vi "ProcCore.vi"(6 "SecondaryData Feed":refnum<queue>, 7 "ProcessParams":T1={"DisplayIncrement"=0, "DisplayIncrementRef"=refnum, "Rep .Rate (Hz)"=10.0, "Save"=FALSE, "SW_Average"=0, "Filter"=enum."None", "FilterParams"=variant, "DAQParams"={"TrigDelay"=0.0, "Offset"=0, "Resolution"=-32768, "Range (mV)"=0, "Sample Rate"=100000000.0, "Depth"=16384.0, "Segments"=1}, "Graph"=[], "CmdParams."=variant, "Average(SW)Ref"=refnum, "Calibr.Params"=refnum, "SignalSegmentRef"=refnum, "WriterQueue"=refnum, "SecData_Interpolation"=FALSE} {"DAQParams"."Segments" min=1 max=1024 step=1; "DAQParams"."Sample Rate" format="%.0p"}, 8 "error in":errorcluster, 9 "Signal buffer in":refnum<queue>, 10 "CtrlQueue in":refnum<queue>) -> (0 "error out":errorcluster)   [LabVIEW 2014]
uses:
  <instrlib>/GenericDAQ/VI/GenericDAQ_Signal.ctl
  ProcessParams.ctl
  ControlDef/ProcessingMode.ctl
  DAQParams.ctl
  DisplayGraph.ctl
  Binning/BinType.ctl
  ControlDef/Average#.ctl
  Files/Signal_Segment.ctl
  ControlDef/Signal.ctl
  ProcessStates.ctl
  <instrlib>/GenericMotionCore/Public/SecondaryDataFeed.ctl
  Binning/SpectrumBinning.vi
  MassResolutionCalc/FindMassResolution_Single.vi
  <instrlib>/GenericMotionCore/GenericMotionCore.lvlib
  <instrlib>/GenericDAQ/GenericDAQ.lvlib
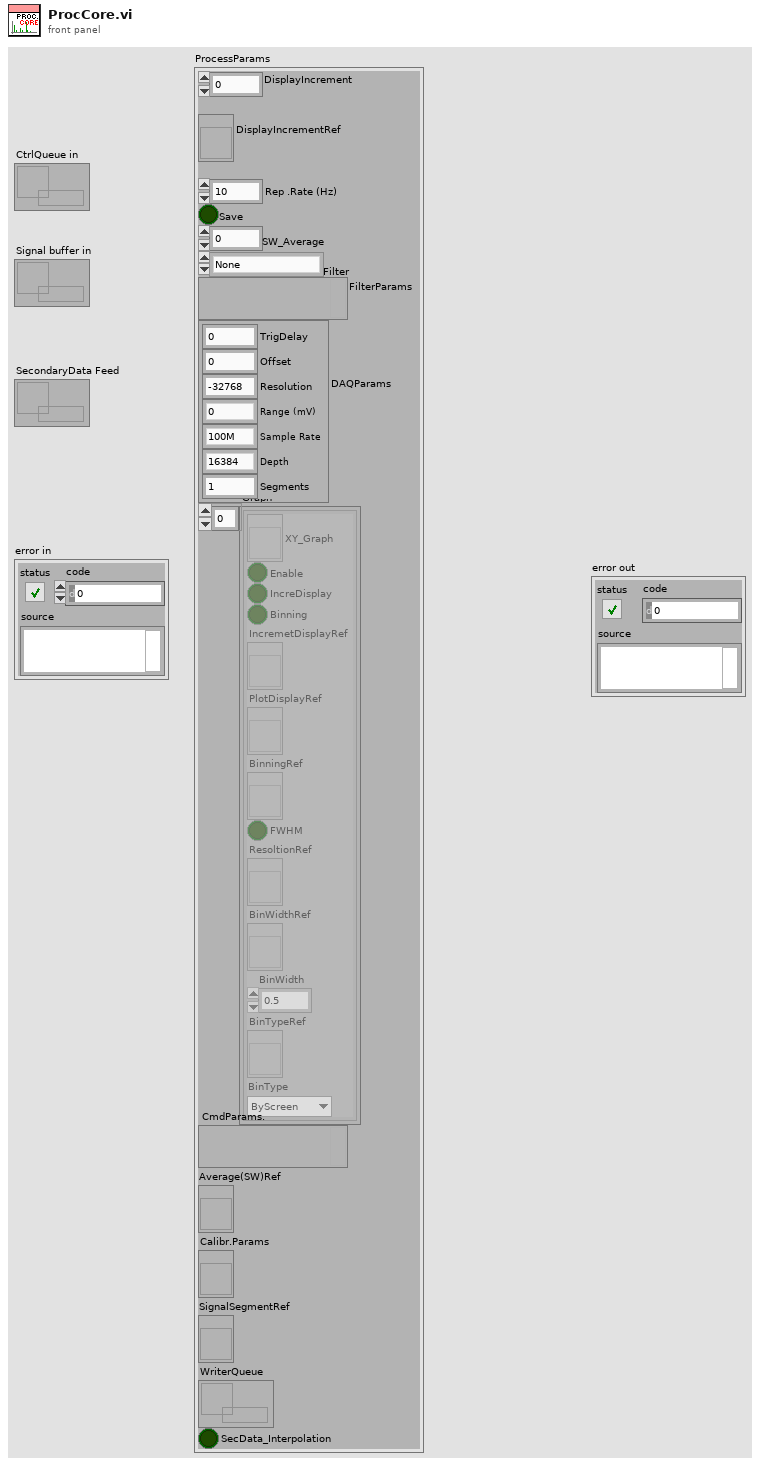
[diagram p1: front panel]
types:
  T1 = typedef "ProcessParams.ctl" = cluster{"DisplayIncrement":u32, "DisplayIncrementRef":refnum<vi>, "Rep .Rate (Hz)":dbl, "Save":bool, "SW_Average":u32, "Filter":T2, "FilterParams":variant, "DAQParams":T3, "Graph":T4[], "CmdParams.":variant, "Average(SW)Ref":refnum<vi>, "Calibr.Params":refnum<vi>, "SignalSegmentRef":refnum<vi>, "WriterQueue":refnum<queue>, "SecData_Interpolation":bool}
  T2 = typedef "ProcessingMode.ctl" = enum16{"None", "Drop by Threshold", "TDC Simulate", "SetFilter"}
  T3 = typedef "DAQParams.ctl" = cluster{"TrigDelay":dbl, "Offset":i32, "Resolution":i32, "Range (mV)":u32, "Sample Rate":dbl, "Depth":dbl, "Segments":u32}
  T4 = typedef "DisplayGraph.ctl" = cluster{"XY_Graph":refnum<vi>, "Enable":bool, "IncreDisplay":bool, "Binning":bool, "IncremetDisplayRef":refnum<vi>, "PlotDisplayRef":refnum<vi>, "BinningRef":refnum<vi>, "FWHM":bool, "ResoltionRef":refnum<vi>, "BinWidthRef":refnum<vi>, "BinWidth":dbl, "BinTypeRef":refnum<vi>, "BinType":T5}
  T5 = typedef "BinType.ctl" = enum16{"ByTime", "ByScreen", "ByMass", "ToUnitMass"}
  T6 = typedef "GenericMotionCore.lvlib/SecondaryDataFeed.ctl" = cluster{"tickcount":u32, "SecondaryData":dbl[]}
  T7 = typedef "ProcessStates.ctl" = enum16{"Initialize", "Normal", "Display", "Write2Buffer", "CalcMzArray", "StartSave", "StopSave", "ConfigChanged", "EndOfLine", "SetFilterParams", "SetGraphsEnable", "SetAcquisitionParams", "ChangeDisplayIncrement", "ChangeRepRate", "SetWriterRef", "Quit", "StartOfLine"}
  T8 = enum16{"Normal", "LineStart", "LineEnd", "FrameStart", "FrameEnd", "Reserved1", "Reserved2"}
  T9 = typedef "GenericDAQ.lvlib/GenericDAQ_Signal.ctl" = cluster{"tickcount":u32, "Signal":sgl[], "SecondaryData":dbl[], "Flag":enum16{"Normal", "LineStart", "LineEnd", "FrameStart", "FrameEnd", "Reserved1", "Reserved2"}, "Segment#":i32}
  T10 = typedef "Signal_Segment.ctl" = cluster{"SampleRate":dbl, "TrigDelay":dbl, "SpecLength":dbl, "DAQ_Range":dbl, "Average#":i32, "Position":dbl[], "Spectrum":sgl[], "Calibr.":dbl[], "Pressure":dbl, "Desp_LaserEnergy":dbl, "PI_LaserEnergy":dbl, "Voltages Table":sgl[][], "ProcMode":T2, "Threshold":dbl, "Comment":string, "TickCount":dbl, "Time Stamp":timestamp}
  T11 = typedef "Average#.ctl" = u16
  T12 = typedef "Signal.ctl" = cluster{"Command":T7, "Params":variant}
  T13 = cluster{"WriterQueue":refnum<queue>, "feedback queue":refnum<queue>}
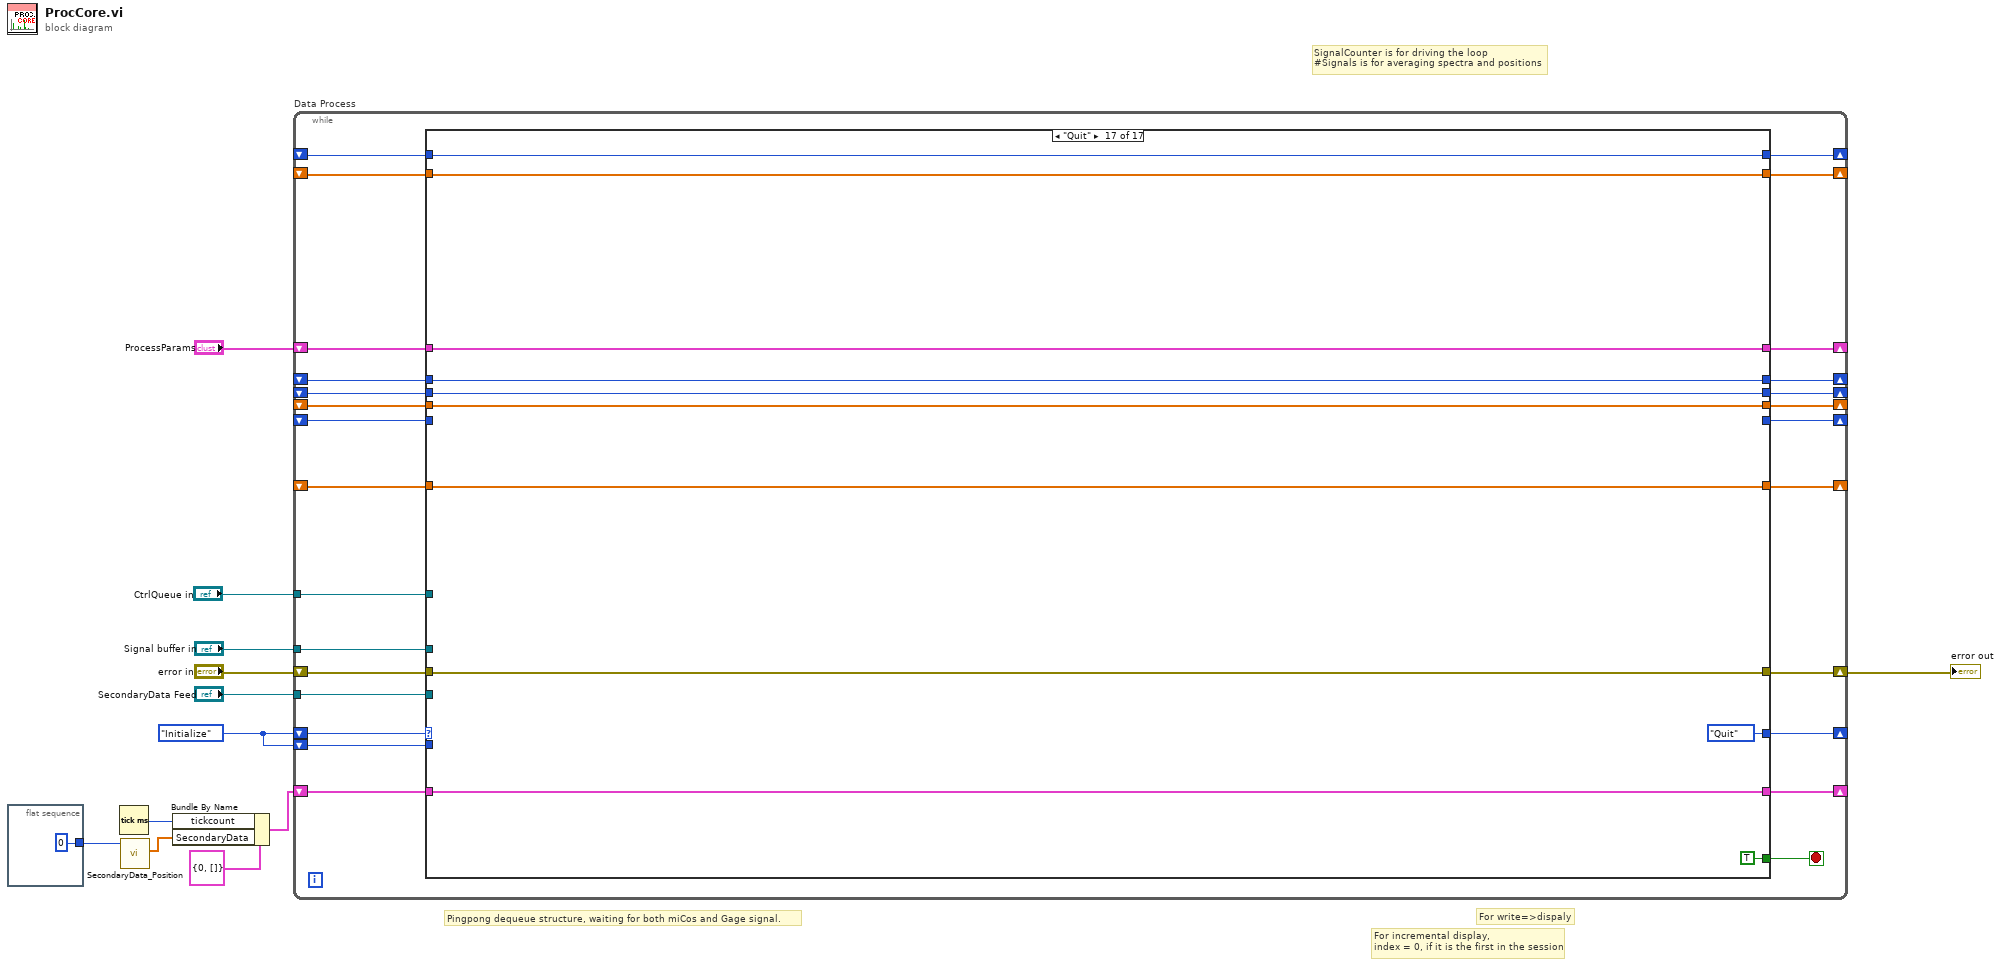
[diagram p0: block diagram]
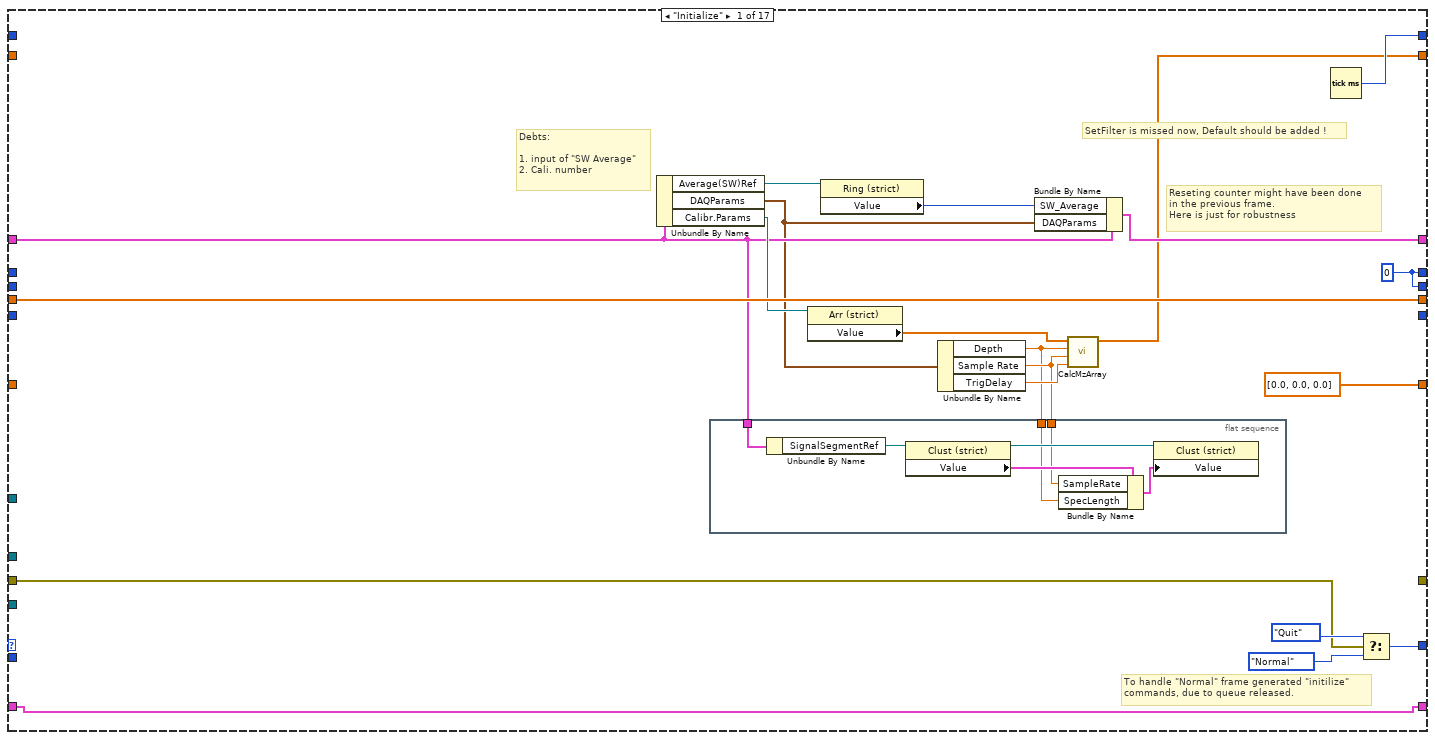
[diagram p2: hidden frame]
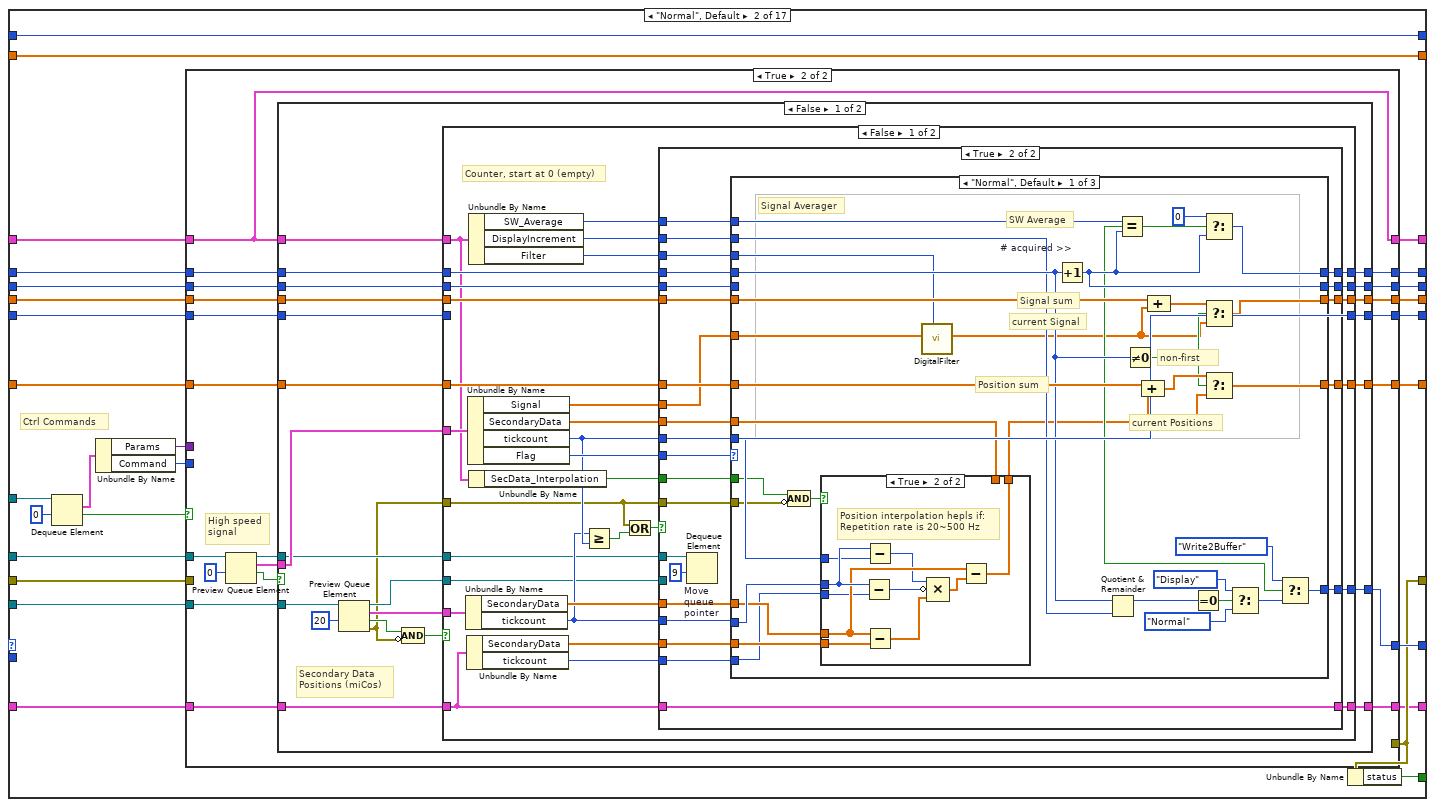
[diagram p3: hidden frame]
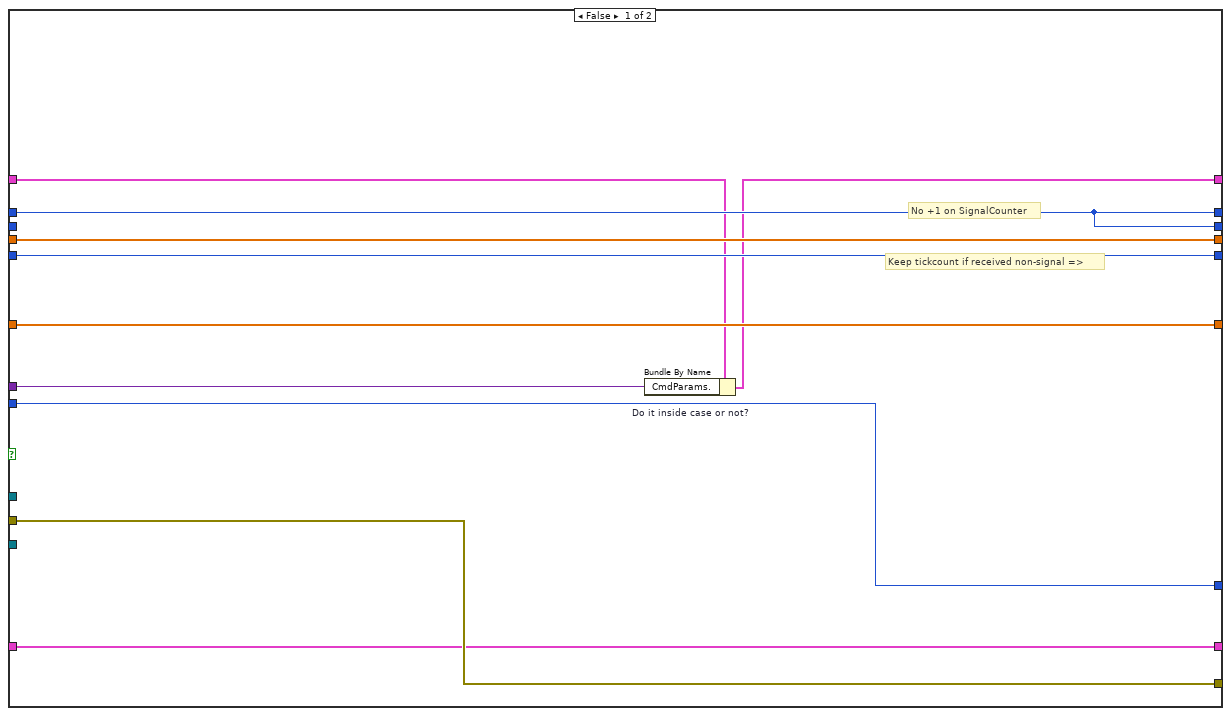
[diagram p4: hidden frame]
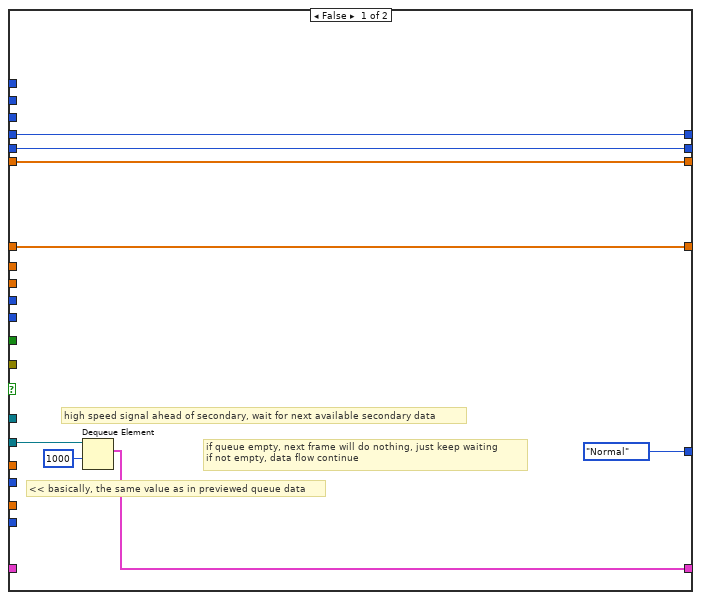
[diagram p5: hidden frame]
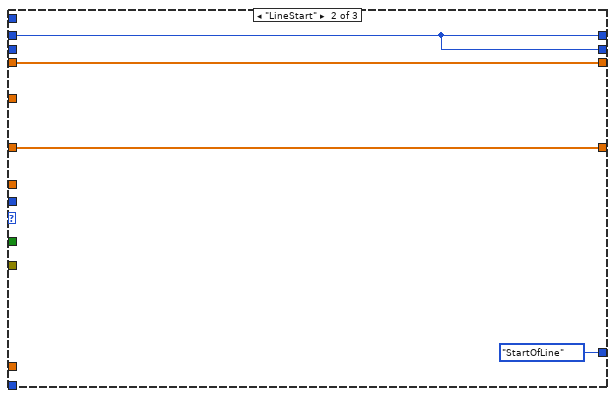
[diagram p7: hidden frame]
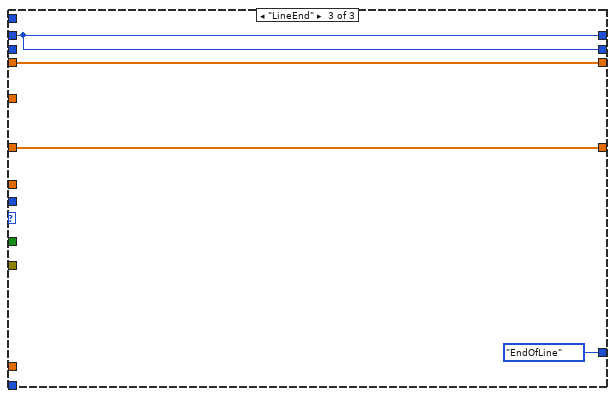
[diagram p8: hidden frame]
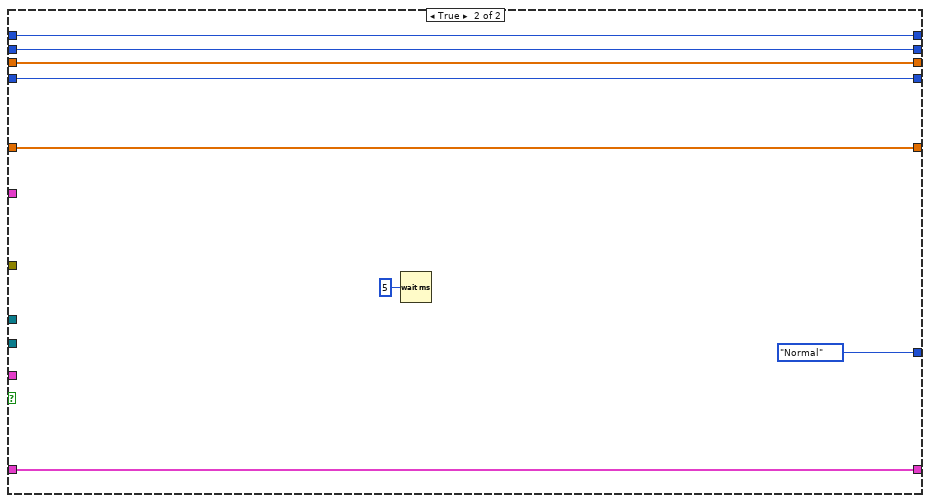
[diagram p9: hidden frame]
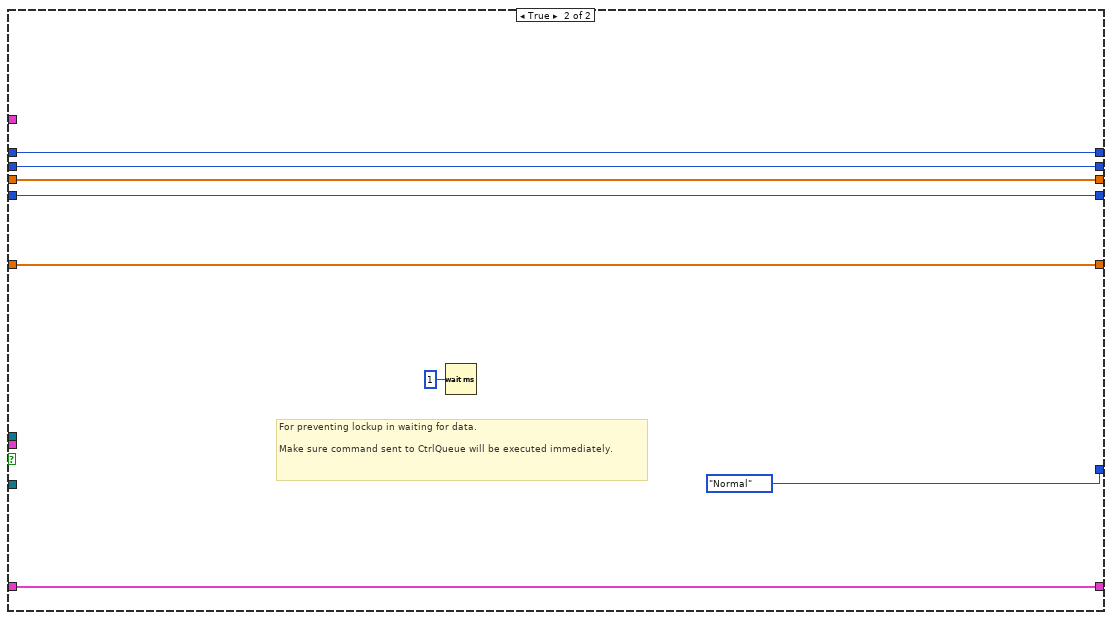
[diagram p10: hidden frame]
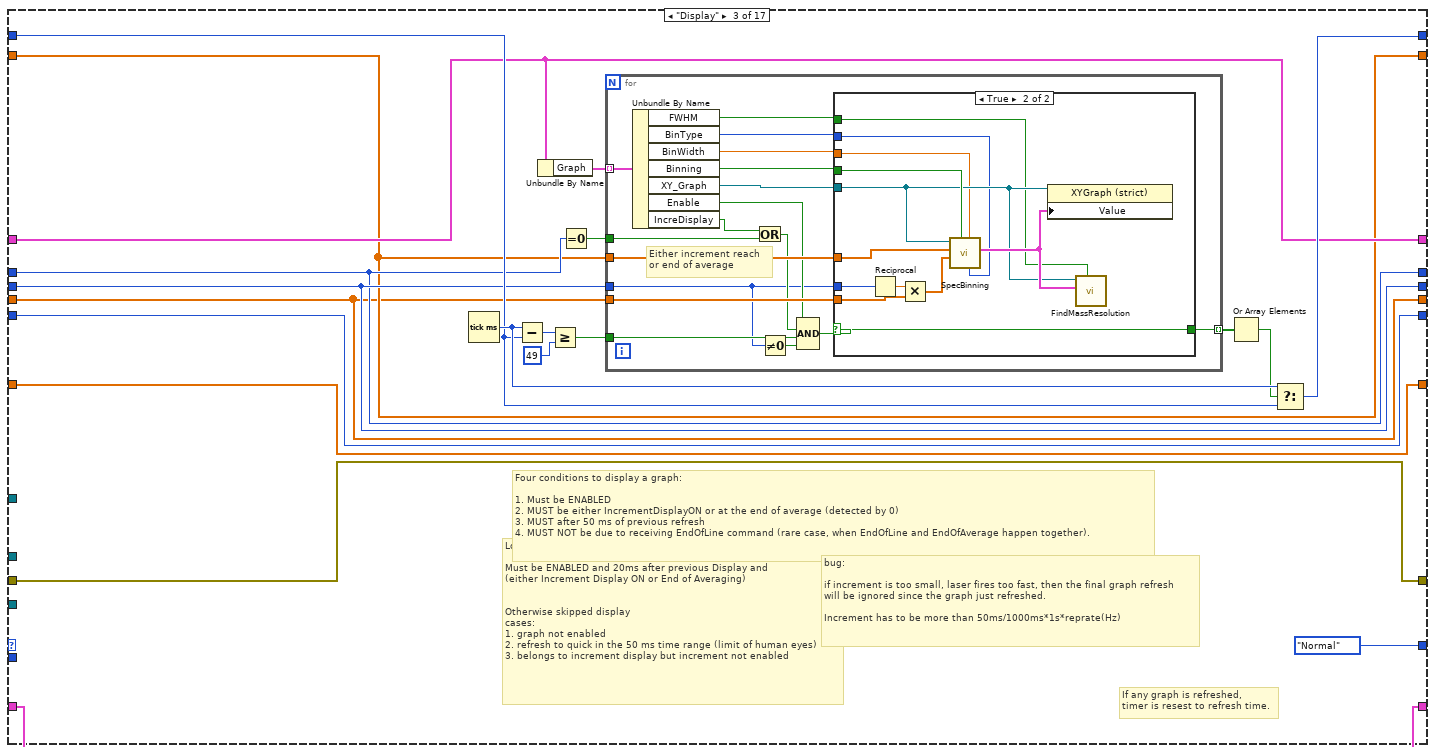
[diagram p11: hidden frame]
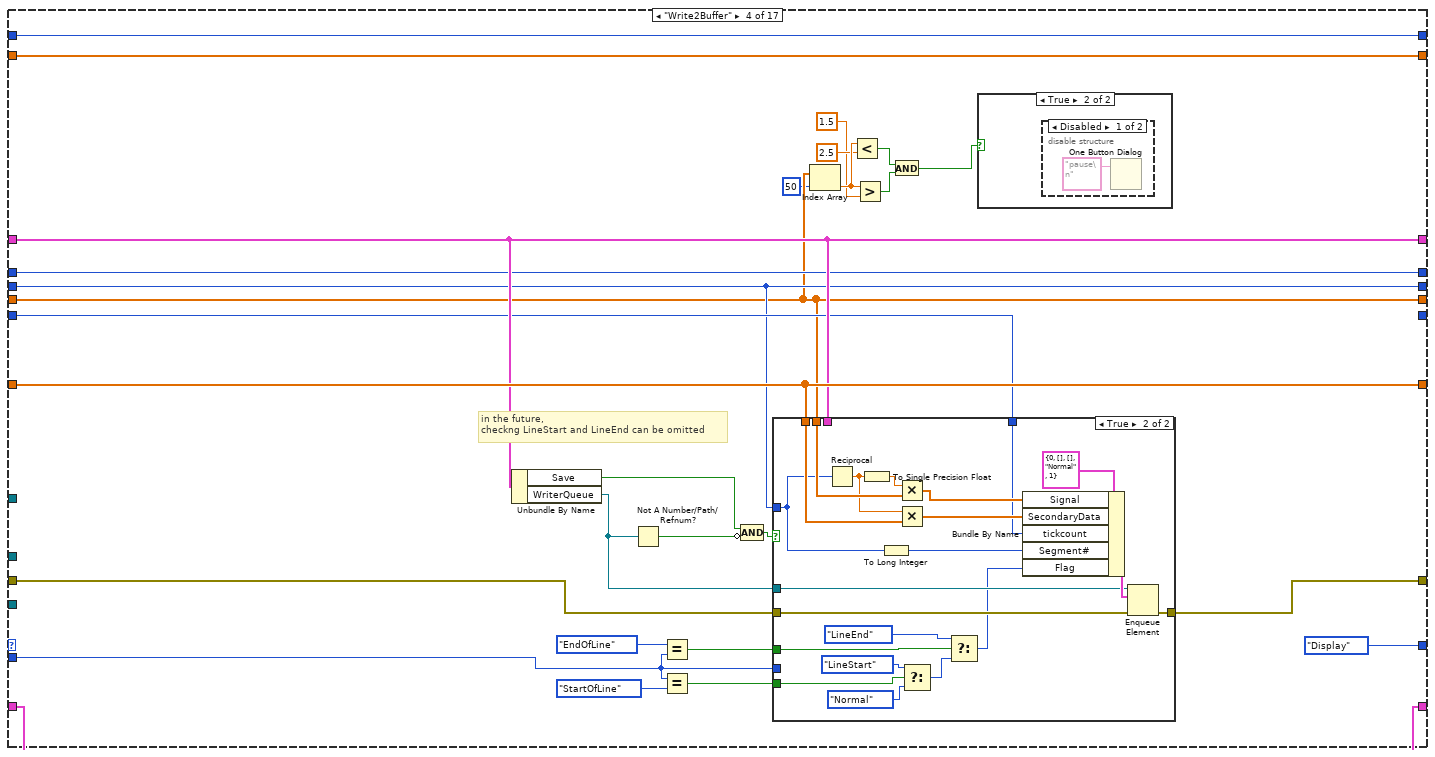
[diagram p13: hidden frame]
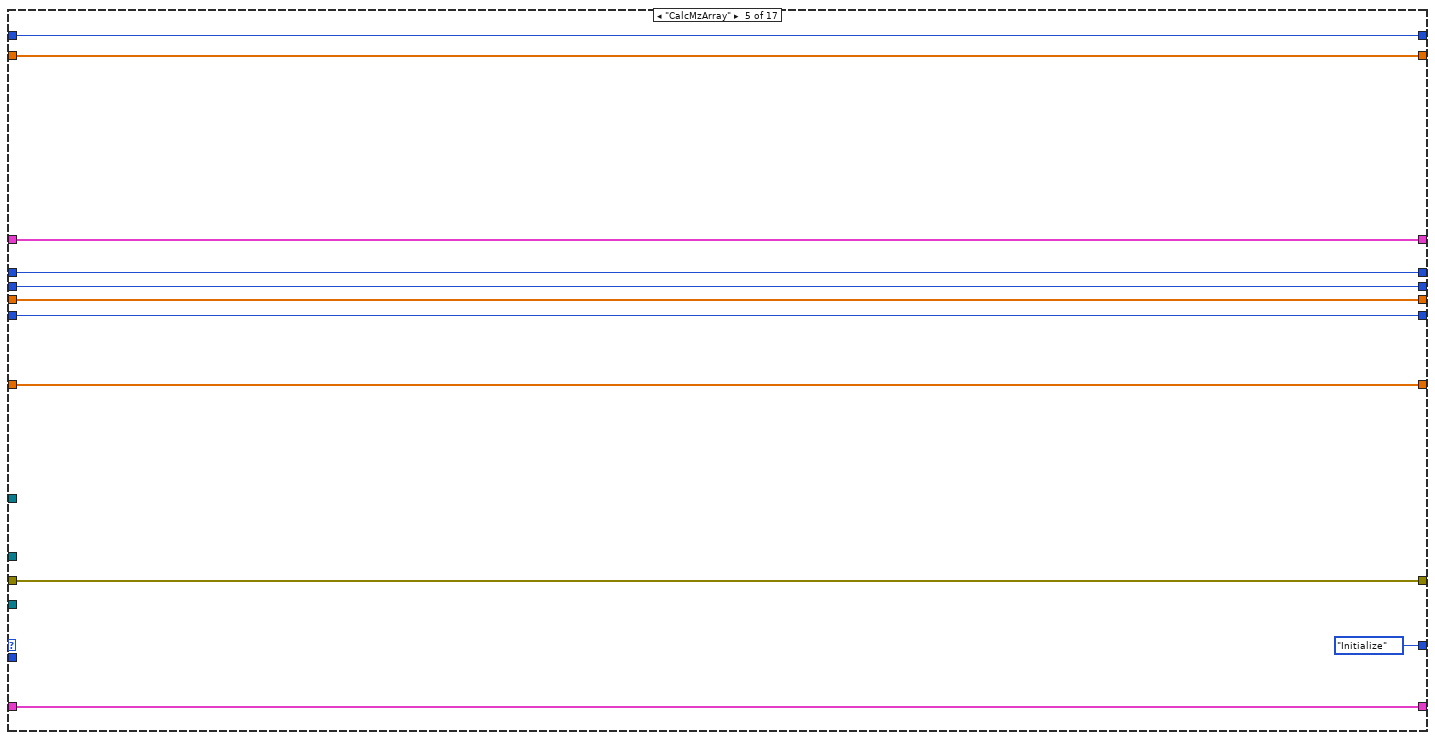
[diagram p17: hidden frame]
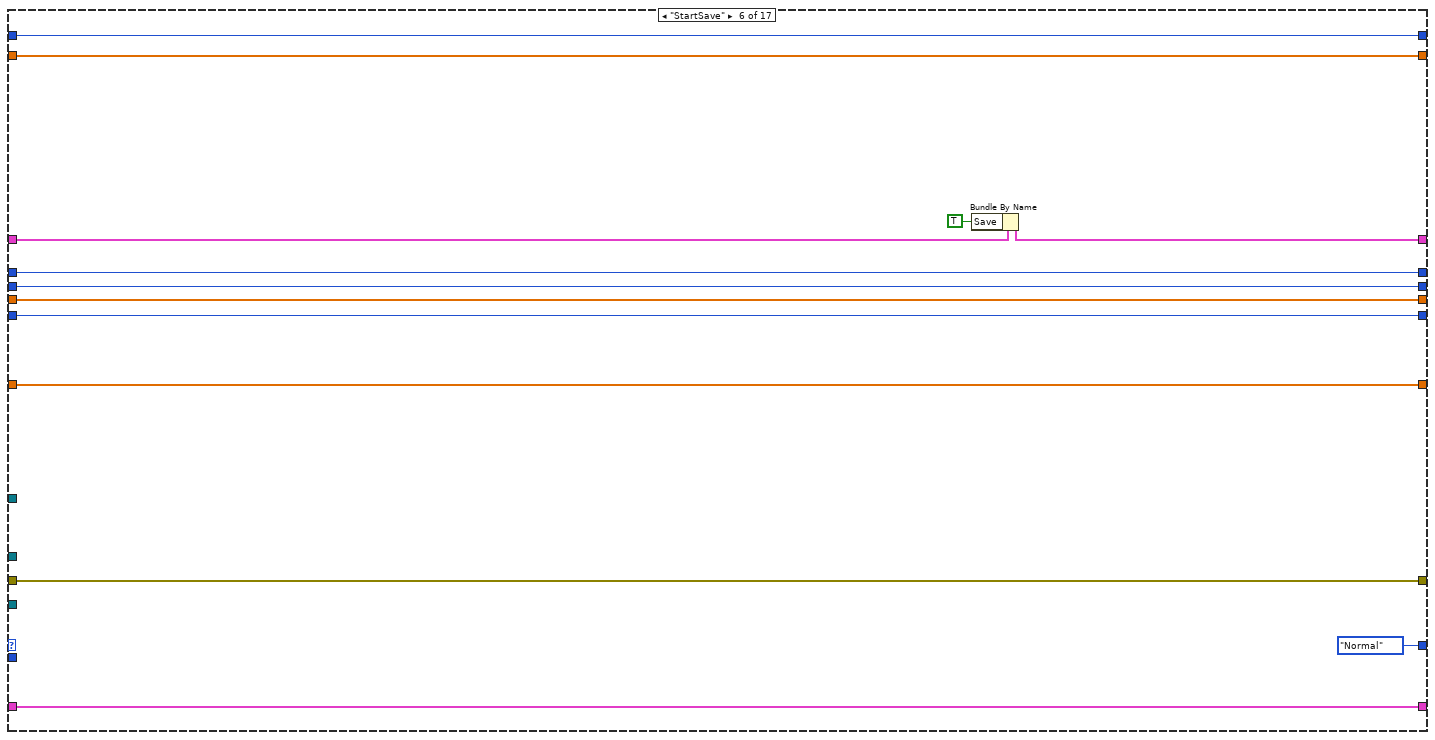
[diagram p18: hidden frame]
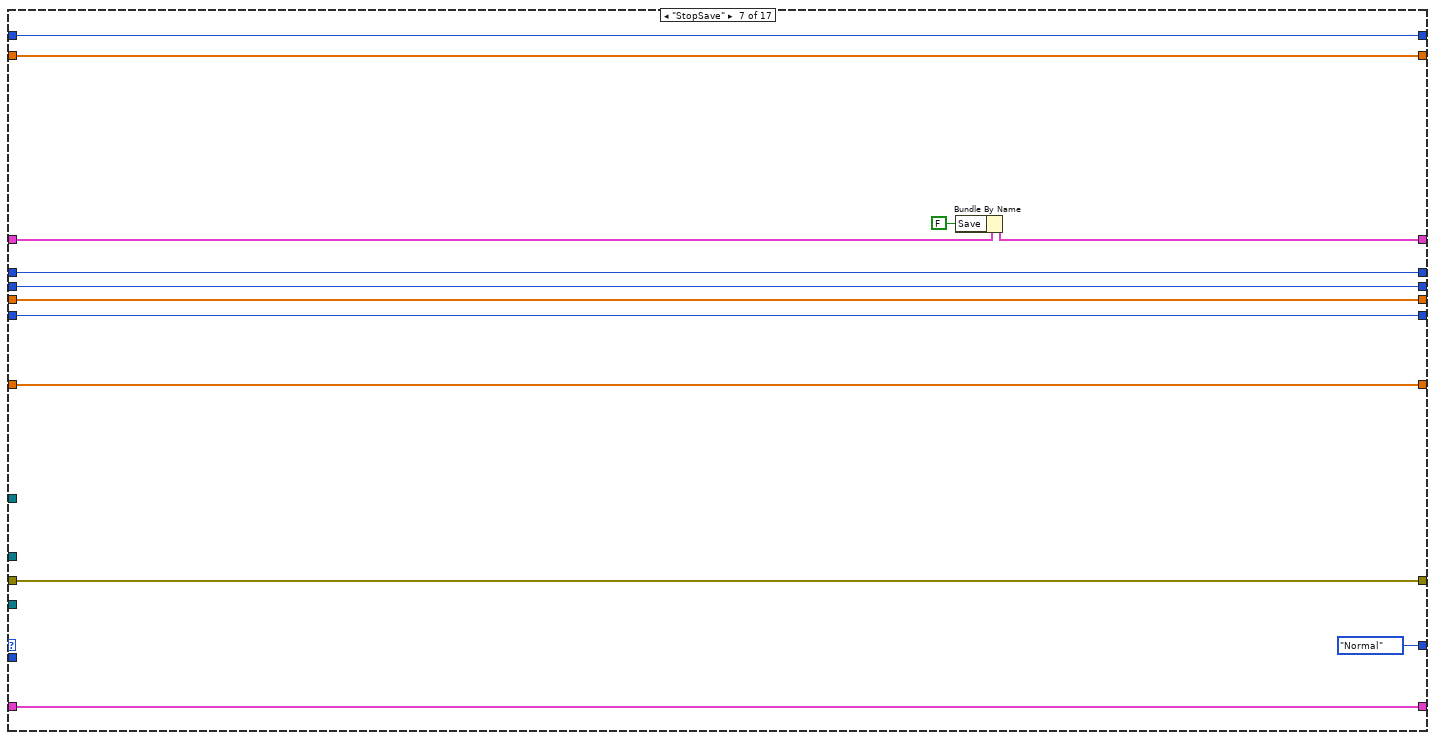
[diagram p19: hidden frame]
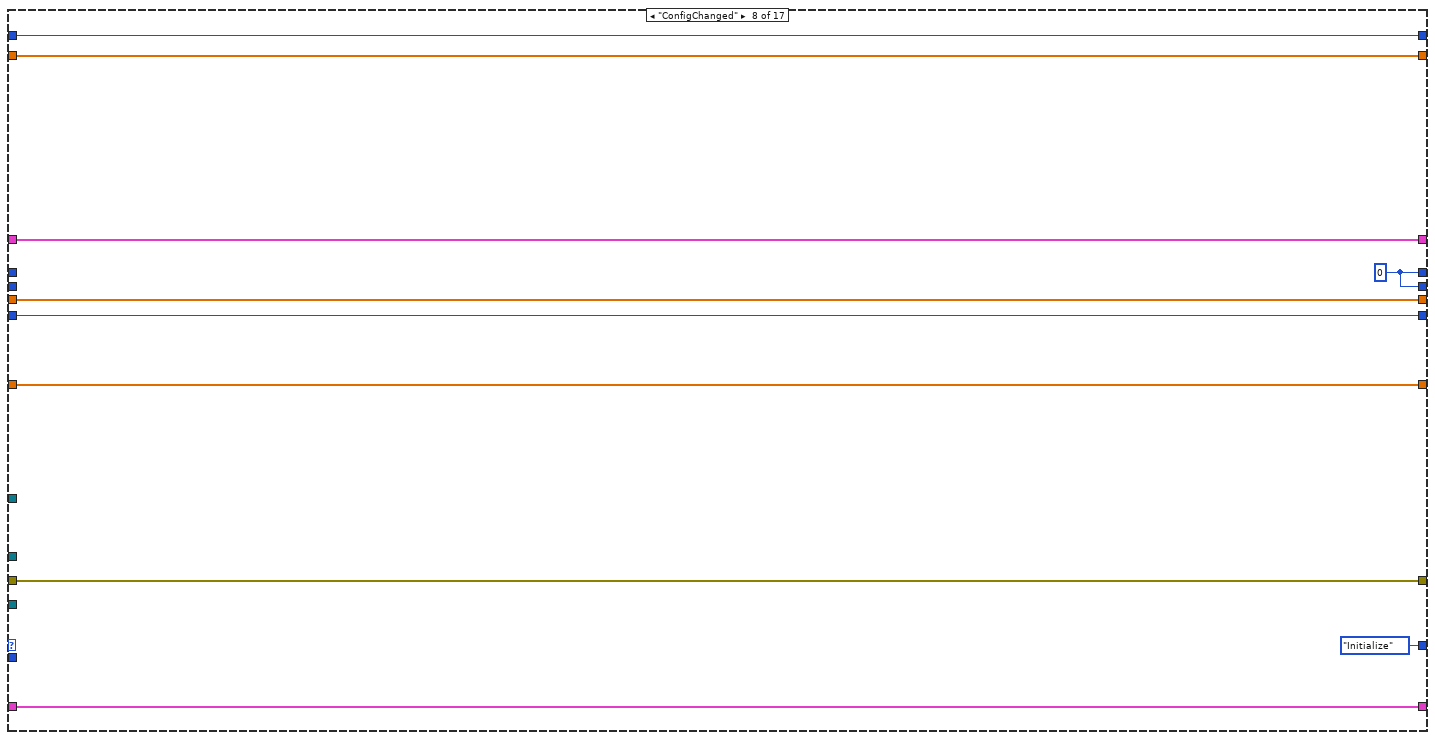
[diagram p20: hidden frame]
diagram:
  w9 = ProcessStates."Initialize"
  # "Pingpong dequeue structure, waiting for both miCos and Gage signal."
  # "For write=>dispaly"
  # "For incremental display,\nindex = 0, if it is the first in the session"
  # "SignalCounter is for driving the loop\n#Signals is for averaging spectra and positions"
  n1 = flat-sequence {
    tunnel: [0 ("Option")] -> w1
    frame #0 {
    }
  }
  n2 = Tick Count (ms)() -> (millisecond timer value=w2:u32)
  n3 = call "SecondaryData_Position.vi"("Option"=w1) -> ("SecondaryData"=w3:dbl[])  [unwired: 10 in]
  n4 = Bundle By Name(cluster=T6 {"tickcount"=0, "SecondaryData"=[]} ("Signal_Typedef"), "tickcount"=w2, "SecondaryData"=w3) -> (w4:T6)
  n5 = while "Data Process" {
    tunnel: "Signal buffer in" -> [w40]
    shift-right: [w34] -> _
    shift-left: _ -> [w38]
    shift-right: [w36] -> _
    shift-left: _ -> [w37]
    shift-right: [w35] -> w10
    shift-left: "error in" -> [w39]
    shift-right: [w26] -> _
    shift-left: _ -> [w32]
    shift-right: [w27] -> _
    shift-left: _ -> [w31]
    shift-right: [w24] -> _
    shift-left: _ -> [w25]
    shift-right: [w29] -> _
    shift-left: "ProcessParams" -> [w30]
    shift-right: [w28] -> _
    shift-left: w9 -> [w23]
    shift-left: w9 -> [w22]
    shift-right: [w21] -> _
    shift-left: _ -> [w20]
    shift-right: [w19] -> _
    shift-left: _ -> [w18]
    tunnel: "CtrlQueue in" -> [w17]
    tunnel: "SecondaryData Feed" -> [w16]
    shift-right: [w15] -> _
    shift-left: w4 -> [w14]
    stop <- w33 stop-if-true
    n6 = case shown="\"Quit\"" w23 {
      tunnel: w40 -> [_ w68 _ _ _ _ _ _ _ _ _ _ _ _ _ _ _]
      tunnel: w39 -> [w48 w76 w301 w356 w391 w404 w417 w427 w438 w449 w466 w480 w501 w534 w561 w585 w608]
      tunnel: w38 -> [w60 w91 w283 w338 w390 w403 w416 w426 w437 w448 w465 w479 w506 w533 w560 w590 w615]
      tunnel: w37 -> [_ w95 w297 w354 w392 w405 w418 w428 w439 w450 w467 w481 w507 w535 w562 w591 w616]
      tunnel: [dbl[] [0.0, 0.0, 0.0] w89 w297 w354 w392 w405 w418 w428 w439 w450 w467 w481 w507 w535 w562 w591 w616] -> w36
      tunnel: [_ w77 w301 w355 w391 w404 w417 w427 w438 w449 w466 w480 w500 w534 w561 w577 w608] -> w35
      tunnel: [w60 w92 w283 w338 w390 w403 w416 w426 w437 w448 w465 w479 w506 w533 w560 w590 w615] -> w34
      tunnel: [_ w86 _ _ _ _ _ _ _ _ _ _ _ _ _ _ TRUE] -> w33
      tunnel: w32 -> [_ w94 w293 w358 w388 w400 w413 w424 w435 w446 w464 w477 w505 w531 w558 w589 w612]
      tunnel: w31 -> [_ w87 w287 w351 w389 w401 w414 _ w432 w443 _ w478 _ w532 w559 _ w613]
      tunnel: w25 -> [_ w93 w284 w357 w385 w399 w412 w423 w434 w445 w463 w476 w504 w530 w557 w588 w611]
      tunnel: w30 -> [w47 w74 w286 w352 w386 w402 w415 w425 w436 w447 w459 w473 w499 w527 w554 w584 w614]
      tunnel: [w56 w73 w286 w352 w386 w398 w411 w425 w436 w447 w462 w475 w502 w526 w549 w586 w614] -> w29
      tunnel: [w49 w90 ProcessStates."Normal" ProcessStates."Display" ProcessStates."Initialize" ProcessStates."Normal" ProcessStates."Normal" ProcessStates."Initialize" ProcessStates."Write2Buffer" ProcessStates."Write2Buffer" ProcessStates."Initialize" ProcessStates."Normal" ProcessStates."Initialize" ProcessStates."Normal" ProcessStates."Normal" ProcessStates."Normal" ProcessStates."Quit"] -> w28
      tunnel: [w44 w88 w287 w351 w389 w401 w414 w421 u32 0 ("t") u32 0 ("t") w453 w478 w498 w532 w559 w583 w613] -> w27
      tunnel: [w58 w94 w294 w358 w388 w400 w413 w424 w435 w446 w464 w477 w505 w531 w558 w589 w612] -> w26
      tunnel: [w43 w93 w284 w357 w385 w399 w412 w423 w434 w445 w463 w476 w504 w530 w557 w588 w611] -> w24
      tunnel: w22 -> [_ _ _ w345 _ _ _ _ _ _ _ _ _ _ _ _ _]
      tunnel: [w44 w85 w289 w349 w384 w395 w408 w421 w432 w443 w453 w470 w498 w529 w556 w583 w607] -> w21
      tunnel: w20 -> [_ w72 w289 w349 w384 w395 w408 _ _ _ _ w470 _ w529 w556 _ w607]
      tunnel: [_ w84 w285 _ w383 w394 w407 w420 w430 w441 w452 w469 w497 w525 w552 w582 _] -> w19
      tunnel: w18 -> [_ w83 w285 w350 w383 w394 w407 w420 w430 w441 w452 w469 w497 w525 w552 w582 _]
      tunnel: w17 -> [_ w81 _ _ _ _ _ _ _ _ _ _ _ _ _ _ _]
      tunnel: w16 -> [_ w71 _ _ _ _ _ _ _ _ _ _ _ _ _ _ _]
      tunnel: [w41 w70 w282 w341 w382 w393 w406 w419 w429 w440 w451 w468 w496 w516 w542 w571 w606] -> w15
      tunnel: w14 -> [w41 w69 w282 w341 w382 w393 w406 w419 w429 w440 w451 w468 w496 w516 w542 w571 w606]
      frame "Initialize" {
        w44 = u32 0 ("t")
        # "SetFilter is missed now, Default should be added !"
        # "Reseting counter might have been done\nin the previous frame.\nHere is just for robustness"
        # "To handle \"Normal\" frame generated \"initilize\"\ncommands, due to queue released."
        # "Debts:\n\n1. input of \"SW Average\"\n2. Cali. number"
        n7 = Unbundle By Name(w47) -> ("Average(SW)Ref"=w55:refnum<vi>, "DAQParams"=w42:T3, "Calibr.Params"=w52:refnum<vi>)
        n8 = flat-sequence {
          tunnel: w47 -> [w67]
          tunnel: w46 -> [w62]
          tunnel: w45 -> [w61]
          frame #0 {
            n9 = Unbundle By Name(w67) -> ("SignalSegmentRef"=w66:refnum<vi>)
            n10 = property class="Clust (strict)"(reference=w66) -> (reference out=w65:refnum<vi>, "Value"=w64:T10)  [unwired: 1 in, 1 out]
            n11 = Bundle By Name(cluster=w64, "SampleRate"=w62, "SpecLength"=w61) -> (w63:T10)
            n12 = property class="Clust (strict)"(reference=w65, "Value"=w63) -> ()  [unwired: 1 in, 2 out]
          }
        }
        n13 = property class="Arr (strict)"(reference=w52) -> ("Value"=w53:dbl[])  [unwired: 1 in, 2 out]
        n14 = property class="Ring (strict)"(reference=w55) -> ("Value"=w54:T11)  [unwired: 1 in, 2 out]
        n15 = Unbundle By Name(w42) -> ("Depth"=w45:dbl, "Sample Rate"=w46:dbl, "TrigDelay"=w57:dbl)
        n16 = Bundle By Name(cluster=w47, "SW_Average"=w54, "DAQParams"=w42) -> (w56:T1)
        n17 = call "CalcMzArray.vi"("TrigDelay"=w57, "Sample Rate"=w46, "Depth"=w45, "mzCali. (a/b/c)"=w53) -> ("mzArray"=w43:dbl[])  [unwired: 7 in]
        n18 = Tick Count (ms)() -> (millisecond timer value=w58:u32)
        n19 = Select(t=ProcessStates."Quit", s=w48, f=ProcessStates."Normal") -> (s? t:f=w49:T7)
      }
      frame "Normal", Default {
        # "Ctrl Commands"
        # "Normal condition, waiting data coming, choose next frame"
        n20 = Dequeue Element(queue=w81, timeout in ms (-1)=0) -> (element=w80:T12, timed out?=w78:bool)  [unwired: 1 in, 2 out]
        n21 = Unbundle By Name(w80) -> ("Params"=w75:variant, "Command"=w79:T7)
        n22 = case shown="True" w78 {
          tunnel: w95 -> [w105 w125]
          tunnel: [w104 w124] -> w92
          tunnel: w91 -> [w104 w123]
          tunnel: [w103 w120] -> w90
          tunnel: w79 -> [w103 _]
          tunnel: [w105 w122] -> w89
          tunnel: [w102 w121] -> w88
          tunnel: w87 -> [w102 w118]
          tunnel: [w102 w119] -> w85
          tunnel: [w101 w117] -> w84
          tunnel: w83 -> [w101 w115]
          tunnel: w74 -> [w98 w114]
          tunnel: w68 -> [_ w113]
          tunnel: [w100 _] -> w77
          tunnel: w76 -> [w100 _]
          tunnel: w75 -> [w99 _]
          tunnel: [w97 w114] -> w73
          tunnel: w72 -> [_ w116]
          tunnel: w71 -> [_ w107]
          tunnel: [w96 w112] -> w70
          tunnel: w69 -> [w96 w111]
          frame False {
            # "Keep tickcount if received non-signal =>"
            # "No +1 on SignalCounter"
            # "Received command other than signal"
            n23 = Bundle By Name "Do it inside case or not?"(cluster=w98, "CmdParams."=w99) -> (w97:T1)
          }
          frame True {
            # "High speed\nsignal"
            # "Normal condition: summing"
            n24 = Preview Queue Element(queue=w113, timeout in ms (-1)=0) -> (queue out=w106:refnum<queue>, element=w110:T9, timed out?=w108:bool)  [unwired: 1 in, 1 out]
            n25 = case shown="False" w108 {
              tunnel: w125 -> [w148 w277]
              tunnel: [w147 w279] -> w124
              tunnel: w123 -> [w146 w279]
              tunnel: [w145 w277] -> w122
              tunnel: [w144 w278] -> w121
              tunnel: [w143 ProcessStates."Normal"] -> w120
              tunnel: [w142 w276] -> w119
              tunnel: w118 -> [w141 w278]
              tunnel: [w138 w275] -> w117
              tunnel: w110 -> [w140 _]
              tunnel: w114 -> [w139 _]
              tunnel: w116 -> [w136 w276]
              tunnel: w115 -> [w130 w275]
              tunnel: [w129 w274] -> w112
              tunnel: w111 -> [w137 w274]
              tunnel: w107 -> [w134 _]
              tunnel: w106 -> [w128 _]
              frame False {
                # "Secondary Data\nPositions (miCos)"
                n26 = Preview Queue Element(queue=w134, timeout in ms (-1)=20) -> (queue out=w131:refnum<queue>, element=w132:T6, timed out?=w133:bool, error out=w126:errorcluster)  [unwired: 1 in]
                n27 = Compound Arithmetic op=AND(w133, invert w126) -> (w127:bool)
                n28 = case shown="False" w127 {
                  tunnel: w148 -> [w179 w270]
                  tunnel: [w178 w271] -> w147
                  tunnel: w146 -> [w177 w271]
                  tunnel: [w176 w270] -> w145
                  tunnel: [w175 w273] -> w144
                  tunnel: [w174 ProcessStates."Normal"] -> w143
                  tunnel: [w173 w272] -> w142
                  tunnel: w141 -> [w172 w273]
                  tunnel: w140 -> [w154 _]
                  tunnel: w139 -> [w150 _]
                  tunnel: [w161 w268] -> w138
                  tunnel: w137 -> [w156 w267]
                  tunnel: w136 -> [w163 w272]
                  tunnel: w132 -> [w162 _]
                  tunnel: w131 -> [w157 _]
                  tunnel: w130 -> [_ w268]
                  tunnel: [w155 w267] -> w129
                  tunnel: w128 -> [w153 _]
                  tunnel: w126 -> [w151 _]
                  frame False {
                    # "Counter, start at 0 (empty)"
                    n29 = Unbundle By Name(w162) -> ("SecondaryData"=w159:dbl[], "tickcount"=w158:u32)
                    n30 = Unbundle By Name(w156) -> ("SecondaryData"=w165:dbl[], "tickcount"=w164:u32)
                    n31 = Unbundle By Name(w154) -> ("Signal"=w170:sgl[], "SecondaryData"=w171:dbl[], "tickcount"=w161:u32, "Flag"=w166:T8)
                    n32 = Unbundle By Name(w150) -> ("SW_Average"=w167:u32, "DisplayIncrement"=w169:u32, "Filter"=w168:T2)
                    n33 = Unbundle By Name(w150) -> ("SecData_Interpolation"=w149:bool)
                    n34 = Greater Or Equal?(x=w158, y=w161) -> (x >= y?=w160:bool)
                    n35 = Or(x=w151, y=w160) -> (x .or. y?=w152:bool)
                    n36 = case shown="True" w152 {
                      tunnel: w179 -> [w182 w212]
                      tunnel: [w183 w211] -> w178
                      tunnel: w177 -> [w183 w210]
                      tunnel: [w182 w209] -> w176
                      tunnel: [w185 w208] -> w175
                      tunnel: [ProcessStates."Normal" w207] -> w174
                      tunnel: [w184 w206] -> w173
                      tunnel: w172 -> [w185 w205]
                      tunnel: w171 -> [_ w204]
                      tunnel: w170 -> [_ w203]
                      tunnel: w169 -> [_ w202]
                      tunnel: w168 -> [_ w201]
                      tunnel: w167 -> [_ w200]
                      tunnel: w166 -> [_ w199]
                      tunnel: w165 -> [_ w198]
                      tunnel: w164 -> [_ w197]
                      tunnel: w163 -> [w184 w196]
                      tunnel: w161 -> [_ w195]
                      tunnel: w159 -> [_ w194]
                      tunnel: w158 -> [_ w193]
                      tunnel: w157 -> [w187 _]
                      tunnel: w156 -> [_ w191]
                      tunnel: [w181 w191] -> w155
                      tunnel: w153 -> [_ w192]
                      tunnel: w151 -> [_ w190]
                      tunnel: w149 -> [_ w188]
                      frame False {
                        # "<< basically, the same value as in previewed queue data"
                        # "if queue empty, next frame will do nothing, just keep waiting\nif not empty, data flow continue"
                        # "high speed signal ahead of secondary, wait for next available secondary data"
                        n37 = Dequeue Element(queue=w187, timeout in ms (-1)=1000) -> (element=w181:T6)  [unwired: 1 in, 3 out]
                      }
                      frame True {
                        n38 = Dequeue Element "Move \nqueue\npointer"(queue=w192, timeout in ms (-1)=9) -> ()  [unwired: 1 in, 4 out]
                        n39 = case shown="\"Normal\", Default" w199 {
                          tunnel: w212 -> [w246 w258 w264]
                          tunnel: [w235 w259 w263] -> w211
                          tunnel: w210 -> [w245 w259 w263]
                          tunnel: [w236 w258 w264] -> w209
                          tunnel: [w244 w260 w262] -> w208
                          tunnel: [w243 ProcessStates."StartOfLine" ProcessStates."EndOfLine"] -> w207
                          tunnel: [w242 w260 w262] -> w206
                          tunnel: w205 -> [w241 w260 w262]
                          tunnel: w204 -> [w218 _ _]
                          tunnel: w203 -> [w240 _ _]
                          tunnel: w202 -> [w239 _ _]
                          tunnel: w201 -> [w238 _ _]
                          tunnel: w200 -> [w237 _ _]
                          tunnel: w193 -> [w234 _ _]
                          tunnel: w195 -> [w233 _ _]
                          tunnel: w194 -> [w231 _ _]
                          tunnel: w198 -> [w232 _ _]
                          tunnel: w197 -> [w230 _ _]
                          tunnel: w196 -> [_ _ _]
                          tunnel: w190 -> [w214 _ _]
                          tunnel: w188 -> [w215 _ _]
                          frame "Normal", Default {
                            # "Signal Averager"
                            # "SW Average"
                            # "non-first"
                            # "Signal sum"
                            # "current Signal"
                            # "Position sum"
                            # "current Positions"
                            n40 = Compound Arithmetic op=AND(w215, invert w214) -> (w216:bool)
                            n41 = case shown="True" w216 {
                              tunnel: w234 -> [_ w257]
                              tunnel: w233 -> [_ w256]
                              tunnel: w232 -> [_ w255]
                              tunnel: w231 -> [_ w254]
                              tunnel: w230 -> [_ w253]
                              tunnel: w218 -> [w247 _]
                              tunnel: [w247 w252] -> w217
                              frame False {
                                # "This frame is for:\n1. MultiRec Mode\n2. Cases neesd no interpolation"
                                # "No interpolation"
                              }
                              frame True {
                                # "Position interpolation hepls if:\nRepetition rate is 20~500 Hz"
                                # "Position Interpolation"
                                n42 = Subtract(x=w257, y=w253) -> (x-y=w250:u32)
                                n43 = Subtract(x=w257, y=w256) -> (x-y=w249:u32)
                                n44 = Subtract(x=w254, y=w255) -> (x-y=w251:dbl[])
                                n45 = Compound Arithmetic op=MULTIPLY(w249, invert w250, w251) -> (w248:dbl[])
                                n46 = Subtract(x=w254, y=w248) -> (x-y=w252:dbl[])
                              }
                            }
                            n47 = call "DigitalFilter.vi"("Filter"=w238, "Original Data"=w240) -> ("Output"=w213:sgl[])  [unwired: 9 in]
                            n48 = Increment "# acquired >>"(x=w241) -> (x+1=w242:u32)
                            n49 = Quotient & Remainder(x=w241, y=w239) -> (x-y*floor(x/y)=w225:u32)  [unwired: 1 out]
                            n50 = Equal?(x=w237, y=w242) -> (x = y?=w223:bool)
                            n51 = Not Equal To 0?(x=w241) -> (x != 0?=w221:bool)
                            n52 = Compound Arithmetic op=ADD(w246, w217) -> (w224:dbl[])
                            n53 = Compound Arithmetic op=ADD(w245, w213) -> (w229:sgl[])
                            n54 = Equal To 0?(x=w225) -> (x = 0?=w226:bool)
                            n55 = Select(t=u32 0, s=w223, f=w242) -> (s? t:f=w244:u32)
                            n56 = Select(t=w229, s=w221, f=w213) -> (s? t:f=w235:sgl[])
                            n57 = Select(t=w224, s=w221, f=w217) -> (s? t:f=w236:dbl[])
                            n58 = Select(t=ProcessStates."Display", s=w226, f=ProcessStates."Normal") -> (s? t:f=w219:T7)
                            n59 = Select(t=ProcessStates."Write2Buffer" ("f"), s=w223, f=w219) -> (s? t:f=w243:T7)
                          }
                          frame "LineStart" {
                          }
                          frame "LineEnd" {
                          }
                        }
                      }
                    }
                  }
                  frame True {
                    n60 = Wait (ms)(milliseconds to wait=u32 5) -> ()  [unwired: 1 out]
                  }
                }
              }
              frame True {
                # "For preventing lockup in waiting for data. \n\nMake sure command sent to CtrlQueue will be executed immediately."
                n61 = Wait (ms)(milliseconds to wait=u32 1) -> ()  [unwired: 1 out]
              }
            }
          }
        }
        n62 = Unbundle By Name(w77) -> ("status"=w86:bool)
      }
      frame "Display" {
        # "bug:\n\nif increment is too small, laser fires too fast, then the final graph refresh\nwill be ignored since the graph just refreshed.\n\nIncrement has to be more than 50ms/1000ms*1s*reprate(Hz)"
        # "Four conditions to display a graph:\n\n1. Must be ENABLED\n2. MUST be either IncrementDisplayON or at the end of average (detected by 0)\n3. MUST after 50 ms of previous refresh\n4. MUST NOT be due to receiving EndOfLine command (rare case, when EndOfLine and EndOfAverage happen together)."
        # "If any graph is refreshed, \ntimer is resest to refresh time."
        # "Logic to Diskplay:\n\nMust be ENABLED and 20ms after previous Display and \n(either Increment Display ON or End of Averaging)\n\n\nOtherwise skipped display\ncases:\n1. graph not enabled\n2. refresh to quick in the 50 ms time range (limit of human eyes)\n3. belongs to increment display but increment not enabled"
        n63 = Tick Count (ms)() -> (millisecond timer value=w295:u32)
        n64 = Subtract(x=w295, y=w293) -> (x-y=w299:u32)
        n65 = Unbundle By Name(w286) -> ("Graph"=w300:T4[])
        n66 = Greater Or Equal?(x=w299, y=u32 49) -> (x >= y?=w296:bool)
        n67 = Equal To 0?(x=w287) -> (x = 0?=w288:bool)
        n68 = for {
          tunnel: w300 -> [w318] mode=indexing
          tunnel: w284 -> [w316]
          tunnel: w283 -> [w315]
          tunnel: w296 -> [w312]
          tunnel: [w309] -> w291 mode=indexing
          tunnel: w289 -> [w305]
          tunnel: w288 -> [w308]
          # "Either increment reach \nor end of average"
          n69 = Unbundle By Name(w318) -> ("FWHM"=w304:bool, "BinType"=w302:T5, "BinWidth"=w303:dbl, "Binning"=w307:bool, "XY_Graph"=w317:refnum<vi>, "Enable"=w313:bool, "IncreDisplay"=w310:bool)
          n70 = Or(x=w310, y=w308) -> (x .or. y?=w311:bool)
          n71 = Not Equal To 0?(x=w305) -> (x != 0?=w306:bool)
          n72 = Compound Arithmetic op=AND(w313, w311, w312, w306) -> (w314:bool)
          n73 = case shown="True" w314 {
            selector: w314 -> [_ w325]
            tunnel: w317 -> [_ w322]
            tunnel: w316 -> [_ w330]
            tunnel: w315 -> [_ w328]
            tunnel: w305 -> [_ w326]
            tunnel: [_ w325] -> w309
            tunnel: w307 -> [_ w324]
            tunnel: w304 -> [_ w321]
            tunnel: w303 -> [_ w320]
            tunnel: w302 -> [_ w319]
            frame False {
            }
            frame True {
              n74 = Reciprocal(x=w326) -> (1/x=w329:dbl)
              n75 = Multiply(x=w329, y=w328) -> (x*y=w327:dbl[])
              n76 = call-poly "SpecBinning.vi"("BinType"=w319, "BinWidth"=w320, "Binning (T)"=w324, "Signal"=w327, "m/z Array"=w330, "GraphRef."=w322) -> ("BinnedSpectrum"=w323:cluster{"m/z Array":dbl[], "Signal":dbl[]})  [unwired: 4 in, 1 out]
              n77 = property class="XYGraph (strict)"(reference=w322, "Value"=w323) -> ()  [unwired: 1 in, 2 out]
              n78 = call-poly "FindMassResolution.vi"("EnableResDisplay"=w321, "BinnedSpectrum"=w323, "GraphRef"=w322) -> ()  [unwired: 7 in, 2 out]
            }
          }
        }
        n79 = Or Array Elements(Boolean array=w291) -> (logical OR=w290:bool)
        n80 = Select(t=w295, s=w290, f=w293) -> (s? t:f=w294:u32)
      }
      frame "Write2Buffer" {
        # "in the future,\ncheckng LineStart and LineEnd can be omitted"
        # "Send averaged spectra to buffer(writer), and continue to graph display"
        n81 = Unbundle By Name(w352) -> ("Save"=w342:bool, "WriterQueue"=w348:refnum<queue>)
        n82 = Not A Number/Path/Refnum?(number/path/refnum=w348) -> (NaN/Path/Refnum?=w343:bool)
        n83 = Equal?(x=ProcessStates."EndOfLine", y=w345) -> (x = y?=w340:bool)
        n84 = Equal?(x=w345, y=ProcessStates."StartOfLine" ("x")) -> (x = y?=w339:bool)
        n85 = Compound Arithmetic op=AND(w342, invert w343) -> (w344:bool)
        n86 = case shown="True" w344 {
          tunnel: w348 -> [_ w380]
          tunnel: w356 -> [w360 w379]
          tunnel: [w360 w378] -> w355
          tunnel: w338 -> [_ w377]
          tunnel: w354 -> [_ w375]
          tunnel: w349 -> [_ w372]
          tunnel: w352 -> [_ _]
          tunnel: w345 -> [_ _]
          tunnel: w350 -> [_ w373]
          tunnel: w340 -> [_ w365]
          tunnel: w339 -> [_ w364]
          frame False {
          }
          frame True {
            n87 = Reciprocal(x=w372) -> (1/x=w361:dbl)
            n88 = To Single Precision Float(number=w361) -> (single precision float=w362:sgl)
            n89 = To Long Integer(number=w372) -> (32bit integer=w363:i32)
            n90 = Multiply(x=w362, y=w377) -> (x*y=w374:sgl[])
            n91 = Multiply(x=w361, y=w375) -> (x*y=w376:dbl[])
            n92 = Select(t=T8."LineStart" ("Flag"), s=w364, f=T8."Normal" ("Flag")) -> (s? t:f=w370:T8)
            n93 = Select(t=T8."LineEnd" ("Flag"), s=w365, f=w370) -> (s? t:f=w366:T8)
            n94 = Bundle By Name(cluster=T9 {"tickcount"=0, "Signal"=[], "SecondaryData"=[], "Flag"=enum."Normal", "Segment#"=1} ("Signal_Typedef"), "Signal"=w374, "SecondaryData"=w376, "tickcount"=w373, "Segment#"=w363, "Flag"=w366) -> (w381:T9)
            n95 = Enqueue Element(queue=w380, element=w381, error in (no error)=w379) -> (error out=w378:errorcluster)  [unwired: 1 in, 2 out]
          }
        }
        n96 = Index Array(array=w338, index=50) -> (element=w336:sgl)
        n97 = Less?(x=w336, y=2.5) -> (x < y?=w332:bool)
        n98 = Greater?(x=w336, y=1.5) -> (0:w333:bool)
        n99 = And(x=w332, y=w333) -> (x .and. y?=w331:bool)
        n100 = case shown="True" w331 {
          frame False {
          }
          frame True {
            n101 = disable-structure shown="Disabled" {
              frame Disabled {
                n102 = One Button Dialog(message="pause\n") -> ()  [unwired: 1 in, 1 out]
              }
              frame Enabled {
              }
            }
          }
        }
      }
      frame "CalcMzArray" {
      }
      frame "StartSave" {
        n103 = Bundle By Name(cluster=w402, "Save"=TRUE) -> (w398:T1)
      }
      frame "StopSave" {
        n104 = Bundle By Name(cluster=w415, "Save"=FALSE) -> (w411:T1)
      }
      frame "ConfigChanged" {
        w421 = u32 0
      }
      frame "EndOfLine" {
        # "SingalCounter should be reset\nfor next round of average"
        # "FlushBuffer, reset averager"
      }
      frame "StartOfLine" {
        # "SingalCounter should be reset\nfor next round of average"
        # "FlushBuffer, reset averager"
      }
      frame "SetFilterParams" {
        w453 = u32 0
        n105 = Unbundle By Name(w459) -> ("CmdParams."=w458:variant)
        n106 = Variant To Data(type=cluster{"Processing Mode":T2, "Variant":variant} {"Processing Mode"=enum."None", "Variant"=variant} ("cluster"), Variant=w458) -> (data=w456:cluster{"Processing Mode":T2, "Variant":variant})  [unwired: 1 in, 1 out]
        n107 = Unbundle(w456) -> ("Processing Mode"=w455:T2, "Variant"=w454:variant)
        n108 = call "DigitalFilter.vi"("Filter"=ProcessingMode."SetFilter", "FilterParams"=w454) -> ()  [unwired: 9 in, 1 out]
        n109 = Bundle By Name(cluster=w459, "Filter"=w455, "FilterParams"=w454) -> (w462:T1)
      }
      frame "SetGraphsEnable" {
        n110 = Unbundle By Name(w473) -> ("Graph"=w472:T4[])
        n111 = for {
          tunnel: w472 -> [w495] mode=indexing
          tunnel: [w488] -> w471 mode=indexing
          n112 = Unbundle By Name(w495) -> ("PlotDisplayRef"=w494:refnum<vi>, "IncremetDisplayRef"=w493:refnum<vi>, "BinningRef"=w492:refnum<vi>, "ResoltionRef"=w486:refnum<vi>, "BinWidthRef"=w484:refnum<vi>, "BinTypeRef"=w483:refnum<vi>)
          n113 = property class="DigNum (strict)"(reference=w484) -> ("Value"=w485:dbl)  [unwired: 1 in, 2 out]
          n114 = property class="Enum (strict)"(reference=w483) -> ("Value"=w482:T5)  [unwired: 1 in, 2 out]
          n115 = property class="Bool (strict)"(reference=w494) -> ("Value"=w491:bool)  [unwired: 1 in, 2 out]
          n116 = property class="Bool (strict)"(reference=w493) -> ("Value"=w490:bool)  [unwired: 1 in, 2 out]
          n117 = property class="Bool (strict)"(reference=w492) -> ("Value"=w489:bool)  [unwired: 1 in, 2 out]
          n118 = property class="Bool (strict)"(reference=w486) -> ("Value"=w487:bool)  [unwired: 1 in, 2 out]
          n119 = Bundle By Name(cluster=w495, "Enable"=w491, "IncreDisplay"=w490, "Binning"=w489, "FWHM"=w487, "BinWidth"=w485, "BinType"=w482) -> (w488:T4)
        }
        n120 = Bundle By Name(cluster=w473, "Graph"=w471) -> (w475:T1)
      }
      frame "SetAcquisitionParams" {
        w498 = u32 0 ("t")
        # "Check compatibility issues between AnalogDiscovery and Gage\n\n\n\nNeed change decision from AnalogDisc to continue here. \nalso, command discovery frame in \"Normal\""
        n121 = disable-structure shown="Enabled" {
          disable-tunnel: [w514 w515] -> w502
          disable-tunnel: w501 -> [w512 _]
          disable-tunnel: [w511 _] -> w500
          disable-tunnel: w499 -> [w510 w515]
          frame Enabled {
            n122 = Unbundle By Name(w510) -> ("DAQParams"=w508:T3, "CmdParams."=w509:variant)
            n123 = Variant To Data(error in=w512, type=w508, Variant=w509) -> (data=w513:T3, error out=w511:errorcluster)
            n124 = Bundle By Name(cluster=w510, "DAQParams"=w513) -> (w514:T1)
          }
          frame Disabled {
          }
        }
      }
      frame "ChangeDisplayIncrement" {
        # "DisplayIncrement has to have a fail-safe value, such as 50"
        # "Should add increment range check \n\nincrement has to be larger than 50/1000*reprate(Hz)"
        n125 = Unbundle By Name(w527) -> ("Rep .Rate (Hz)"=w524:dbl, "DisplayIncrementRef"=w519:refnum<vi>, "DisplayIncrement"=w517:u32)
        n126 = property class="DigNum (strict)"(reference=w519) -> (reference out=w520:refnum<vi>, "Value"=w518:u32)  [unwired: 1 in, 1 out]
        n127 = Multiply(x=0.049, y=w524) -> (x*y=w522:dbl)
        n128 = Greater?(x=w518, y=w522) -> (0:w521:bool)
        n129 = case "Bug: actually, not working" shown="True" w521 {
          tunnel: w527 -> [w538 w541]
          tunnel: [w538 w540] -> w526
          tunnel: w518 -> [_ w539]
          tunnel: w520 -> [w537 _]
          tunnel: w517 -> [w536 _]
          frame False {
            n130 = property class="DigNum (strict)"(reference=w537, "Value"=w536) -> ()  [unwired: 1 in, 2 out]
          }
          frame True {
            n131 = Bundle By Name(cluster=w541, "DisplayIncrement"=w539) -> (w540:T1)
          }
        }
      }
      frame "ChangeRepRate" {
        n132 = Unbundle By Name(w554) -> ("DisplayIncrementRef"=w543:refnum<vi>, "DisplayIncrement"=w546:u32, "CmdParams."=w550:variant)
        n133 = Variant To Data(type=0.0 ("Rep .Rate (Hz)"), Variant=w550) -> (data=w544:dbl)  [unwired: 1 in, 1 out]
        n134 = Bundle By Name(cluster=w554, "Rep .Rate (Hz)"=w544) -> (w553:T1)
        n135 = Multiply(x=0.049, y=w544) -> (x*y=w547:dbl)
        n136 = Greater?(x=w547, y=w546) -> (0:w545:bool)
        n137 = case shown="True" w545 {
          tunnel: w553 -> [w563 w570]
          tunnel: [w563 w569] -> w549
          tunnel: w544 -> [_ w568]
          tunnel: w543 -> [_ w566]
          frame False {
          }
          frame True {
            n138 = Divide(x=w568, y=10.0) -> (x/y=w565:dbl)
            n139 = Round Toward +Infinity(x=w565) -> (ceil(x): smallest int >= x=w564:dbl)
            n140 = property class="DigNum (strict)"(reference=w566, "Value"=w564) -> ()  [unwired: 1 in, 2 out]
            n141 = Bundle By Name(cluster=w570, "DisplayIncrement"=w564) -> (w569:T1)
          }
        }
      }
      frame "SetWriterRef" {
        w583 = u32 0 ("t")
        n142 = flat-sequence {
          tunnel: [w605] -> w586
          tunnel: w585 -> [w597]
          tunnel: w584 -> [w604]
          tunnel: [w598] -> w581
          tunnel: [w593] -> w574
          tunnel: [w592] -> w573
          frame #0 {
            n143 = Unbundle By Name(w604) -> ("WriterQueue"=w600:refnum<queue>, "CmdParams."=w601:variant)
            n144 = Bundle("WriterQueue"=w600, "feedback queue"=refnum<queue> refnum) -> (w603:T13)  [unwired: 1 in]
            n145 = Variant To Data(error in=w597, type=w603, Variant=w601) -> (data=w602:T13, error out=w593:errorcluster)
            n146 = Variant To Data(error in=w597, type=w600, Variant=w601) -> (data=w596:refnum<queue>, error out=w592:errorcluster)
            n147 = Unbundle(w602) -> ("WriterQueue"=w595:refnum<queue>, "feedback queue"=w598:refnum<queue>)
            n148 = Select(t=w595, s=w592, f=w596) -> (s? t:f=w594:refnum<queue>)
            n149 = Bundle By Name(cluster=w604, "WriterQueue"=w594) -> (w605:T1)
          }
        }
        n150 = Merge Errors(w574, w573) -> (w572:errorcluster)
        n151 = And(x=w574, y=w573) -> (x .and. y?=w575:bool)
        n152 = Enqueue Element(queue=w581, element="SetWriter_Done", error in (no error)=w574) -> (error out=w578:errorcluster)  [unwired: 1 in, 2 out]
        n153 = call <vilib>:"Clear Errors.vi"("error in (no error)"=w578, "specific error code to clear (0: all)"=91 ("[exception code]")) -> ("error out"=w576:errorcluster)  [unwired: 4 in, 1 out]
        n154 = Select(t=w572, s=w575, f=w576) -> (s? t:f=w577:errorcluster)
      }
      frame "Quit" {
      }
    }
  }
  "error out" <- w10
